vi "RH_SCOPE_Configure.vi"(6 "Digital Trigger?":bool=TRUE, 7 "SCOPE Global Parameters":T2={"min sample rate"=20000000.0, "min record length"=1000, "reference position"=5.0, "input impedance"=0, "maximum input frequency"=0.0, "vertical coupling"=1, "vertical range"=10.0, "vertical offset"=0.0, "NumRecords"=0} {"maximum input frequency" format="%.2f"; "input impedance" items=["1 mega ohm"=0, "50 ohms"=2]; "vertical offset" format="%.4f"; "vertical range" format="%.2f"; "vertical coupling" items=["AC", "DC", "Ground"]; "reference position" format="%#_13g"; "min sample rate" format="%^.2e"}, 8 "error in":errorcluster, 9 "trigger source":T1="VAL_RTSI_0", 10 "channels":string="0", 11 "SCOPE Session In":refnum<k15>) -> (0 "error out":errorcluster, 3 "SCOPE Session Out":refnum<k15>)   [LabVIEW 2023, in "ResourceHandling.lvlib"]
doc: "Configure the Scope session"
uses:
  ResourceHandling.lvlib
  TypeDefs/RH_SCOPE_Parameters.ctl
  <instrlib>/niScope/Controls/niScope vertical coupling.ctl
  <instrlib>/niScope/Controls/niScope trigger source digital.ctl
  <instrlib>/niScope/Configure/Trigger/niScope Configure Trigger Digital.vi
  <instrlib>/niScope/Configure/Trigger/niScope Configure Trigger Immediate.vi
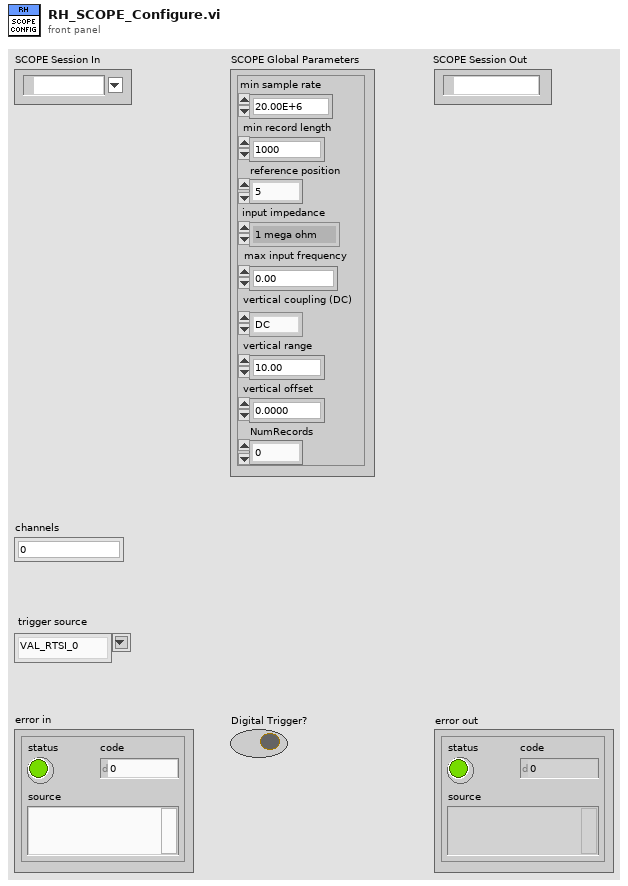
[diagram p1: front panel]
types:
  T1 = typedef "niScope trigger source digital.ctl" = string
  T2 = typedef "ResourceHandling.lvlib/RH_SCOPE_Parameters.ctl" = cluster{"min sample rate":dbl, "min record length":i32, "reference position":dbl, "input impedance":u32, "maximum input frequency":dbl, "vertical coupling":T3, "vertical range":dbl, "vertical offset":dbl, "NumRecords":i32}
  T3 = typedef "niScope vertical coupling.ctl" = i32
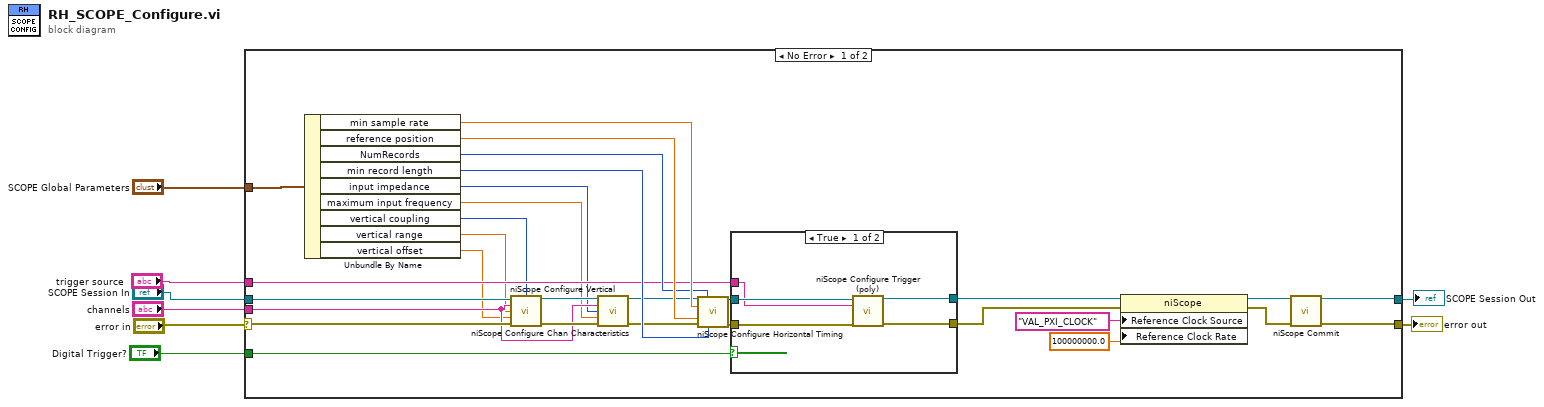
[diagram p0: block diagram]
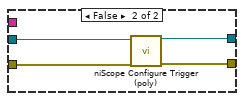
[diagram p2: hidden frame]
diagram:
  n1 = case shown="No Error" "error in" {
    selector: "error in" -> [w20 w47]
    tunnel: "SCOPE Global Parameters" -> [w37 _]
    tunnel: "SCOPE Session In" -> [w19 w48]
    tunnel: [w15 w47] -> w7
    tunnel: [w14 w48] -> w2
    tunnel: "Digital Trigger?" -> [w28 _]
    tunnel: "trigger source" -> [w25 _]
    tunnel: "channels" -> [w18 _]
    frame No Error {
      n2 = Unbundle By Name(w37) -> ("min sample rate"=w34:dbl, "reference position"=w33:dbl, "NumRecords"=w26:i32, "min record length"=w27:i32, "input impedance"=w13:u32, "maximum input frequency"=w12:dbl, "vertical coupling"=w11:T3, "vertical range"=w10:dbl, "vertical offset"=w9:dbl)
      n3 = call <instrlib>:"niScope Configure Vertical.vi"("instrument handle"=w19, "vertical coupling"=w11, "channels"=w18, "vertical range"=w10, "vertical offset"=w9, "error in"=w20) -> ("instrument handle out"=w24:refnum<k15>, "error out"=w21:errorcluster)  [unwired: 8 in]
      n4 = call <instrlib>:"niScope Configure Chan Characteristics.vi"("instrument handle"=w24, "channels"=w18, "input impedance"=w13, "maximum input frequency"=w12, "error in"=w21) -> ("instrument handle out"=w22:refnum<k15>, "error out"=w23:errorcluster)  [unwired: 9 in]
      n5 = call <instrlib>:"niScope Configure Horizontal Timing.vi"("instrument handle"=w22, "number of records"=w26, "min sample rate"=w34, "reference position"=w33, "error in"=w23, "min record length"=w27) -> ("instrument handle out"=w36:refnum<k15>, "error out"=w35:errorcluster)  [unwired: 8 in]
      n6 = case shown="True" w28 {
        tunnel: w36 -> [w42 w46]
        tunnel: w35 -> [w41 w45]
        tunnel: [w40 w44] -> w32
        tunnel: [w39 w43] -> w31
        tunnel: w25 -> [w38 _]
        frame True {
          n7 = call-poly <instrlib>:"niScope Configure Trigger (poly).vi"("instrument handle"=w42, "trigger source"=w38, "error in"=w41) -> ("instrument handle out"=w40:refnum<k15>, "error out"=w39:errorcluster)  [unwired: 11 in]
        }
        frame False {
          n8 = call-poly <instrlib>:"niScope Configure Trigger (poly).vi"("instrument handle"=w46, "error in"=w45) -> ("instrument handle out"=w44:refnum<k15>, "error out"=w43:errorcluster)  [unwired: 12 in]
        }
      }
      n9 = property class="niScope"(reference=w32, error in=w31, "Reference Clock Source"="VAL_PXI_CLOCK" ("Clocking:Reference (Input) Clock Source"), "Reference Clock Rate"=100000000.0 ("Clocking:Reference Clock Rate")) -> (reference out=w17:refnum<k15>, error out=w16:errorcluster)
      n10 = call <instrlib>:"niScope Commit.vi"("instrument handle"=w17, "error in"=w16) -> ("instrument handle out"=w14:refnum<k15>, "error out"=w15:errorcluster)  [unwired: 12 in]
    }
    frame Error {
    }
  }
  "error out" <- w7
  "SCOPE Session Out" <- w2
